vi "PCert-ConfigPageNF-CloseDBConn.vi"(8 "error in (no error)":errorcluster, 11 "ERP-ConfigPageNF in":refnum<class "PCert-ConfigPageNF.lvclass">) -> (0 "error out":errorcluster, 3 "ERP-ConfigPageNF out":refnum<class "PCert-ConfigPageNF.lvclass">)   [LabVIEW 2013, in "PCert-ConfigPageNF.lvclass"]
uses:
  PCert-ConfigPageNF.lvclass
  PCert-ConfigPageNF.lvclass/PCert-ConfigPageNF.ctl
  ftw-dataflow/Actor/src/Connector/FTW-ActorConnector.lvclass
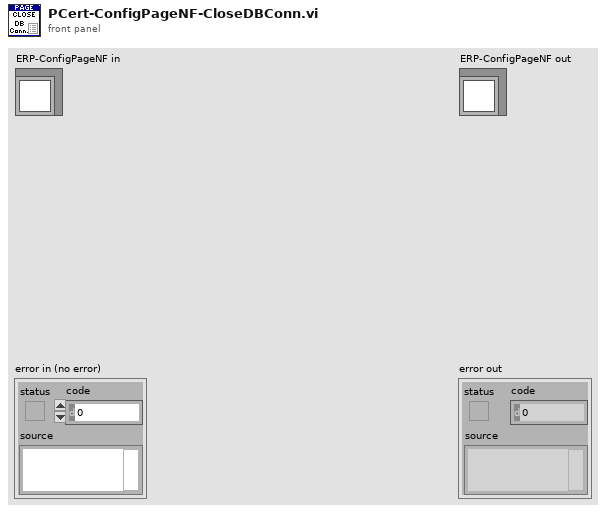
[diagram p1: front panel]
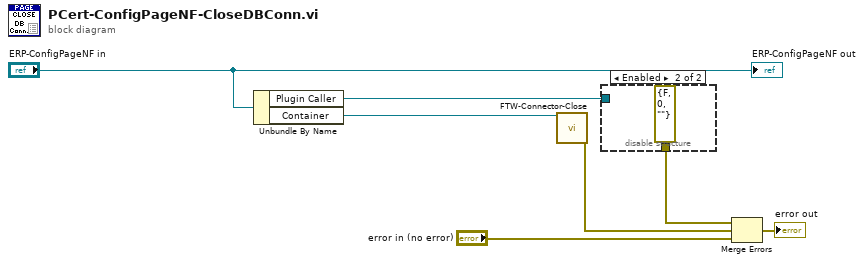
[diagram p0: block diagram]
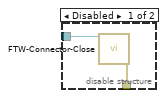
[diagram p2: hidden frame]
diagram:
  n1 = Unbundle By Name("ERP-ConfigPageNF in") -> ("Plugin Caller"=w5:refnum<class "FTW-ActorConnector.lvclass">, "Container"=w6:refnum<class "FTW-ActorConnector.lvclass">)
  n2 = call-dynamic "FTW-Connector-Close.vi"("FTW Actor Connector"=w6) -> ("error out"=w3:errorcluster)  [unwired: 14 in]
  n3 = disable-structure shown="Enabled" {
    disable-tunnel: w5 -> [w9 _]
    disable-tunnel: [w8 errorcluster {"status"=FALSE, "code"=0, "source"=""} ("error out")] -> w2
    frame Disabled {
      n4 = call-dynamic "FTW-Connector-Close.vi"("FTW Actor Connector"=w9) -> ("error out"=w8:errorcluster)  [unwired: 14 in]
    }
    frame Enabled {
    }
  }
  n5 = Merge Errors(w2, w3, "error in (no error)") -> (→"error out":errorcluster)
  "ERP-ConfigPageNF out" <- "ERP-ConfigPageNF in"
